vi "Wait(ms).vi"(8 "error in (no error)":errorcluster, 11 "milliseconds":u32) -> (0 "error out":errorcluster)   [LabVIEW 2015, in "Tool Interface.lvlib"]
uses:
  Tool Interface.lvlib
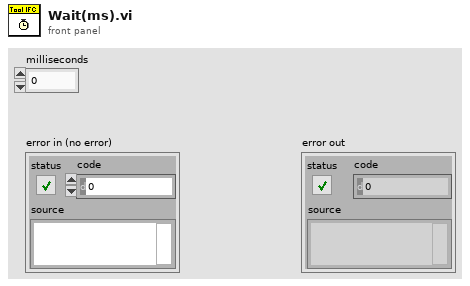
[diagram p1: front panel]
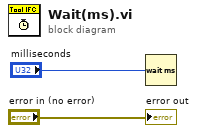
[diagram p0: block diagram]
diagram:
  n1 = Wait (ms)(milliseconds to wait="milliseconds") -> ()  [unwired: 1 out]
  "error out" <- "error in (no error)"
